vi "Test_QMH_Timer.vi"(8 "error in (no error)":errorcluster caption="entrée d'erreur (pas d'erreur)", 11 "Queue TIMER":refnum<queue>) -> (0 "error out":errorcluster caption="sortie d'erreur")   [LabVIEW 2015]
uses:
  controls/QMH_Pirenea_MessageCluster.ctl
panel:
  out "Remaining Time":string
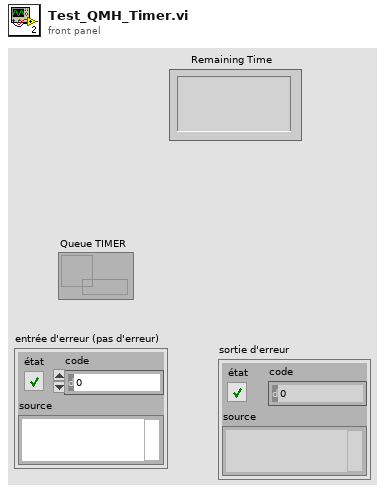
[diagram p1: front panel]
types:
  T1 = typedef "QMH_Pirenea_MessageCluster.ctl" = cluster{"Command":enum16{"Initialize", "Load", "Settings", "Save", "Start", "Stop", "Exit"}, "Data":variant}
  T2 = typedef "QMH_Pirenea_MessageCluster.ctl" = cluster{"Command":enum16{"Initialize", "Start Measure", "Start Same Measure", "Start Next Measure", "Stop Measure", "Write Data", "Measure is Finished", "Emergency Stop", "Exit"}, "Data":variant}
  T3 = enum16{"Initialize", "Start Measure", "Start Same Measure", "Start Next Measure", "Stop Measure", "Write Data", "Measure is Finished", "Emergency Stop", "Exit"}
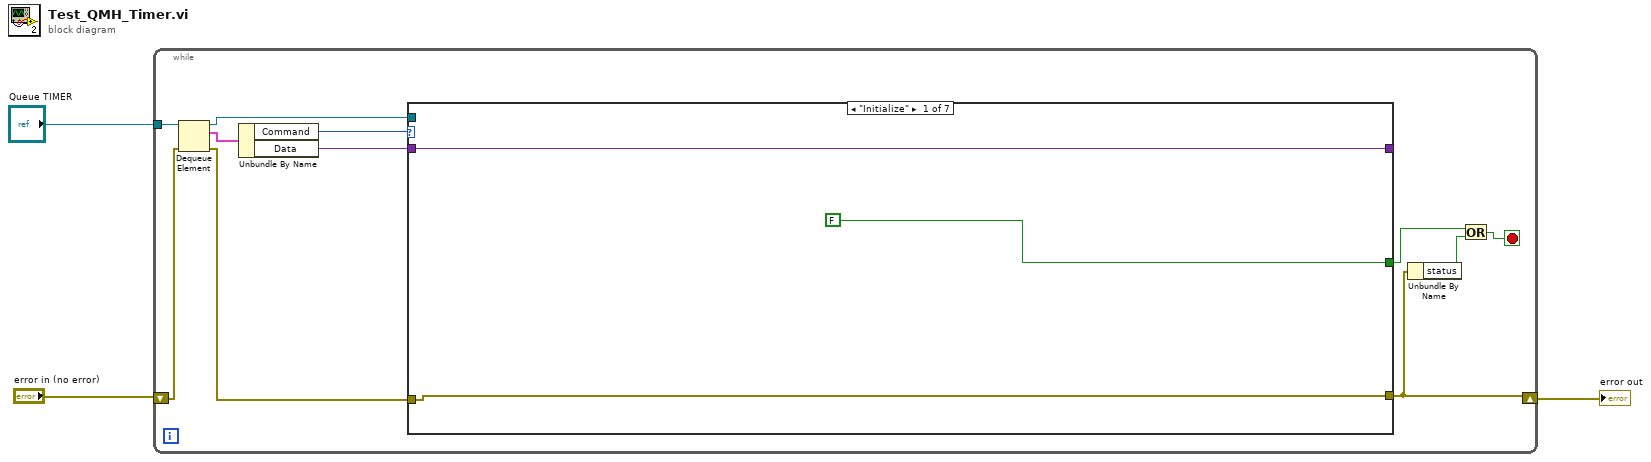
[diagram p0: block diagram]
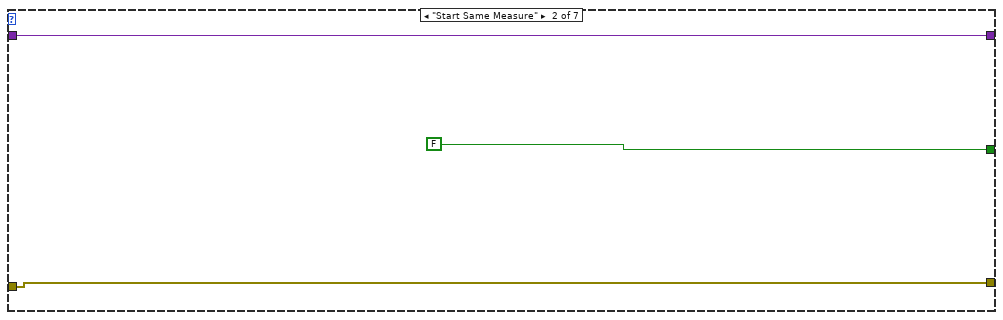
[diagram p2: hidden frame]
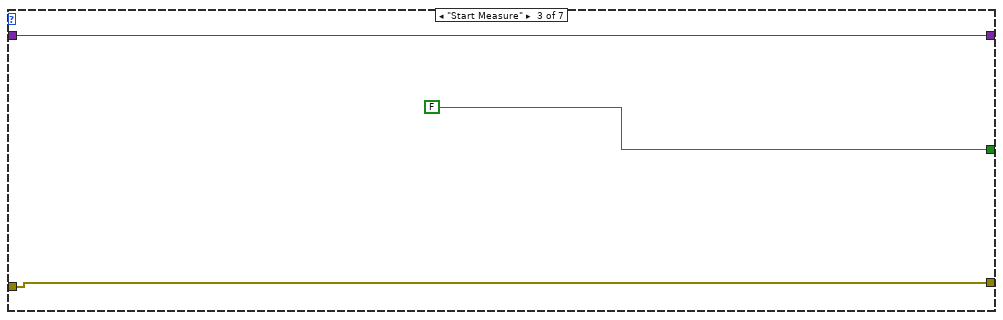
[diagram p3: hidden frame]
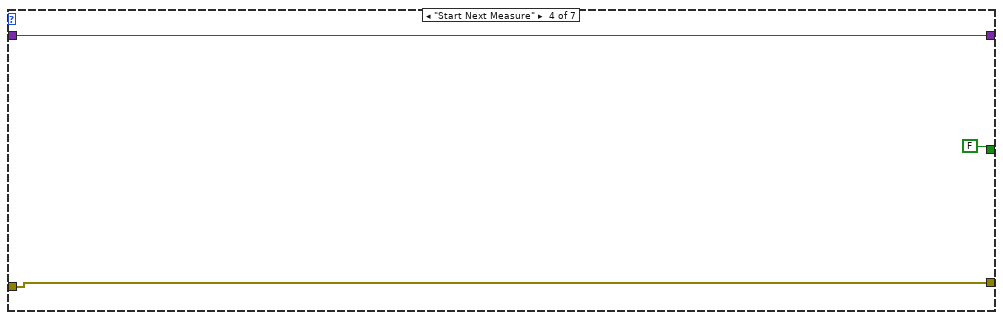
[diagram p4: hidden frame]
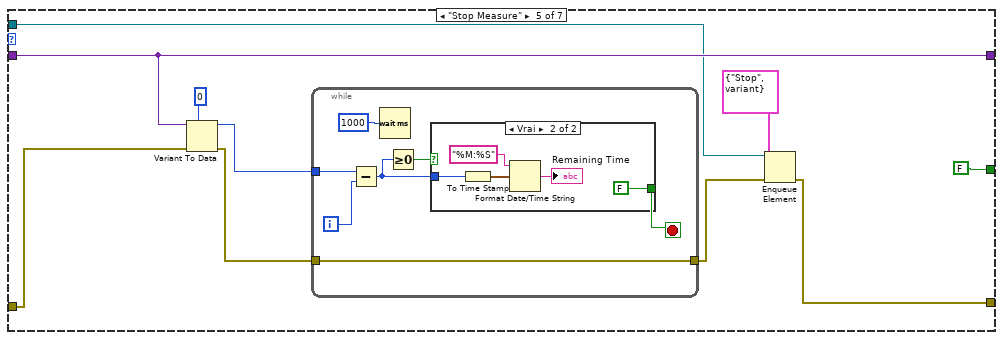
[diagram p5: hidden frame]
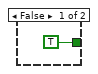
[diagram p6: hidden frame]
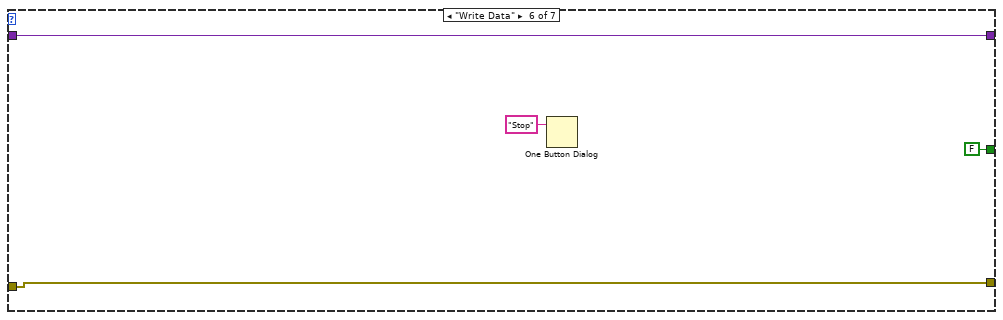
[diagram p7: hidden frame]
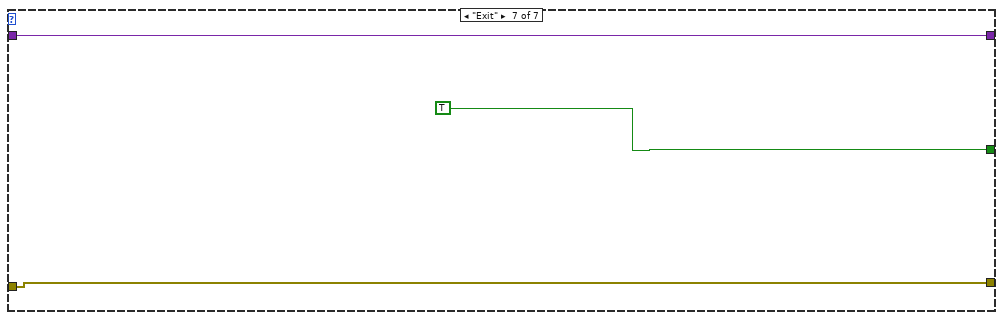
[diagram p8: hidden frame]
diagram:
  n1 = while {
    tunnel: "Queue TIMER" -> [w14]
    shift-right: [w4] -> w1
    shift-left: "error in (no error)" -> [w7]
    stop <- w10 stop-if-true
    n2 = Dequeue Element(queue=w14, error in (no error)=w7) -> (queue out=w5:refnum<queue>, element=w11:T2, error out=w6:errorcluster)  [unwired: 2 out]
    n3 = Unbundle By Name(w11) -> ("Command"=w8:T3, "Data"=w9:variant)
    n4 = case shown="\"Initialize\"" w8 {
      tunnel: [w16 w19 w22 w26 w34 w52 w55] -> _
      tunnel: [FALSE ("x") FALSE ("x") FALSE ("x") FALSE ("x") FALSE ("x") FALSE ("x") TRUE ("x")] -> w12
      tunnel: w9 -> [w16 w19 w22 w26 w34 w52 w55]
      tunnel: w6 -> [w15 w18 w21 w24 w33 w50 w54]
      tunnel: w5 -> [_ _ _ _ w29 _ _]
      tunnel: [w15 w18 w21 w24 w27 w50 w54] -> w4
      frame "Initialize" {
      }
      frame "Start Same Measure" {
      }
      frame "Start Measure" {
      }
      frame "Start Next Measure" {
      }
      frame "Stop Measure" {
        n5 = Variant To Data(error in=w33, type=0, Variant=w34) -> (data=w32:i32, error out=w31:errorcluster)
        n6 = while {
          tunnel: w32 -> [w41]
          tunnel: w31 -> [w37]
          tunnel: [w37] -> w30
          i -> [w42]
          stop <- w38 stop-if-true
          n7 = Subtract(x=w41, y=w42) -> (x-y=w39:i32)
          n8 = Wait (ms)(milliseconds to wait=u32 1000) -> ()  [unwired: 1 out]
          n9 = Greater Or Equal To 0?(x=w39) -> (x >= 0?=w40:bool)
          n10 = case shown="Vrai" w40 {
            tunnel: w39 -> [_ w46]
            tunnel: [TRUE FALSE] -> w38
            frame False {
            }
            frame True {
              n11 = To Time Stamp(1:w46) -> (0:w48:timestamp)
              n12 = Format Date/Time String(time format string (%c)="%M:%S" ("chaîne de format de l'heure (%c)"), seconds (now)=w48) -> (date/time string=→"Remaining Time":string)  [unwired: 1 in]
            }
          }
        }
        n13 = Enqueue Element(queue=w29, element=T1 {"Command"=enum."Stop", "Data"=variant} ("élément"), error in (no error)=w30) -> (error out=w27:errorcluster)  [unwired: 1 in, 2 out]
      }
      frame "Write Data" {
        n14 = One Button Dialog(message="Stop") -> ()  [unwired: 1 in, 1 out]
      }
      frame "Exit" {
      }
    }
    n15 = Unbundle By Name(w4) -> ("status"=w13:bool)
    n16 = Or(x=w12, y=w13) -> (x .or. y?=w10:bool)
  }
  "error out" <- w1
